vi "ReadVolumePoint.vi"(10 "Scan Settings":T1, 11 "Command":enum16{"Init", "Get Point"}(ring)) -> (2 "Finished":bool, 3 "Point":cluster{"X":i32, "Y":i32, "Z":i32})   [LabVIEW 2012]
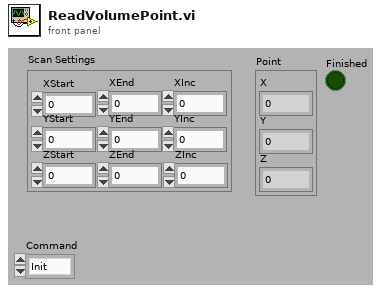
[diagram p1: front panel]
types:
  T1 = cluster{"XStart":i32, "XEnd":i32, "XInc":i32, "YStart":i32, "YEnd":i32, "YInc":i32, "ZStart":i32, "ZEnd":i32, "ZInc":i32}
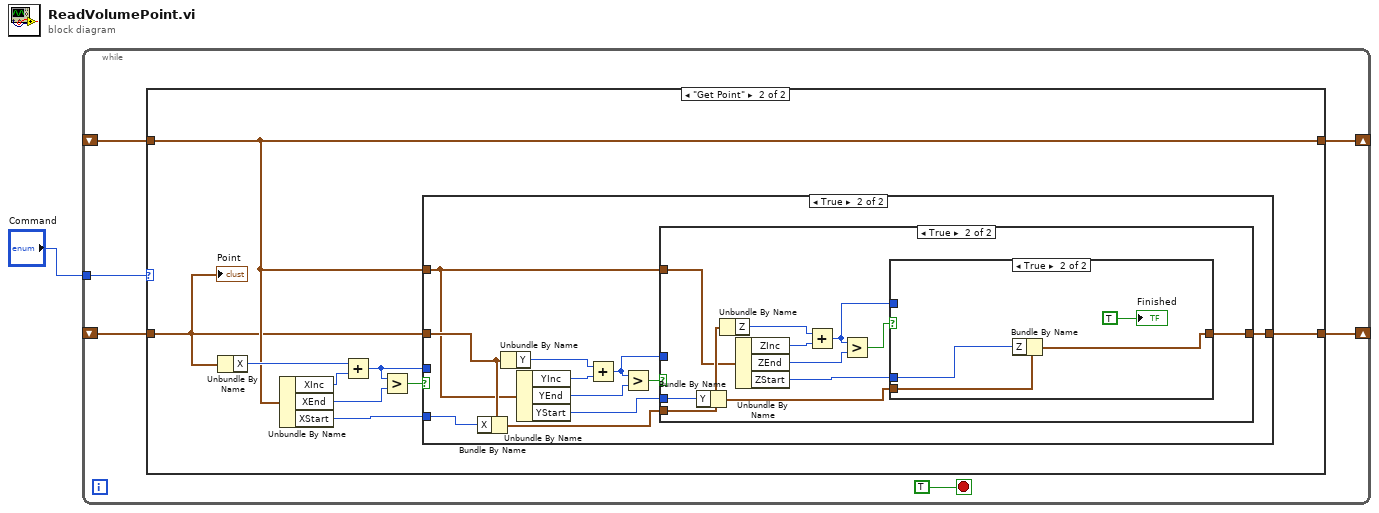
[diagram p0: block diagram]
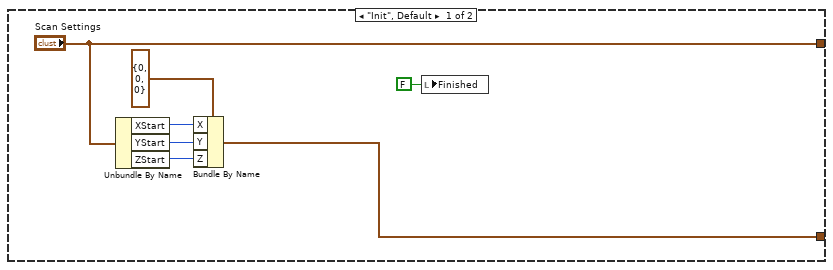
[diagram p2: hidden frame]
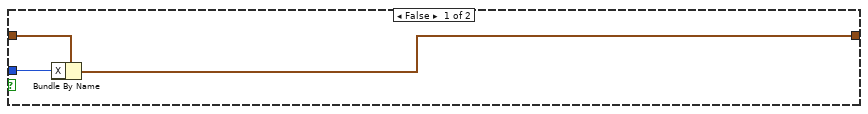
[diagram p3: hidden frame]
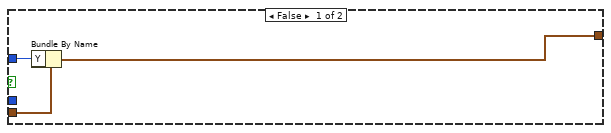
[diagram p4: hidden frame]
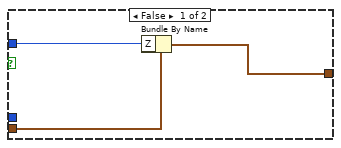
[diagram p5: hidden frame]
diagram:
  n1 = while {
    tunnel: "Command" -> [w6]
    shift-right: [w5] -> _
    shift-left: _ -> [w4]
    shift-right: [w2] -> _
    shift-left: _ -> [w3]
    stop <- TRUE stop-if-true
    n2 = case shown="\"Get Point\"" w6 {
      tunnel: ["Scan Settings" w19] -> w5
      tunnel: w4 -> [_ w19]
      tunnel: w3 -> [_ w17]
      tunnel: [w10 w16] -> w2
      frame "Init", Default {
        n3 = Unbundle By Name("Scan Settings") -> ("XStart"=w13:i32, "YStart"=w12:i32, "ZStart"=w11:i32)
        n4 = Bundle By Name(cluster=cluster{"X":i32, "Y":i32, "Z":i32} {"X"=0, "Y"=0, "Z"=0} ("Point"), "X"=w13, "Y"=w12, "Z"=w11) -> (w10:cluster{"X":i32, "Y":i32, "Z":i32})
        n5 = local write "Finished"(FALSE ("Finished")) -> ()
      }
      frame "Get Point" {
        n6 = Unbundle By Name(w17) -> ("X"=w23:i32)
        n7 = Unbundle By Name(w19) -> ("XInc"=w22:i32, "XEnd"=w21:i32, "XStart"=w15:i32)
        n8 = Add(x=w23, y=w22) -> (x+y=w18:i32)
        n9 = Greater?(x=w18, y=w21) -> (0:w20:bool)
        n10 = case shown="True" w20 {
          tunnel: w19 -> [_ w28]
          tunnel: w18 -> [w25 _]
          tunnel: w17 -> [w26 w37]
          tunnel: [w24 w31] -> w16
          tunnel: w15 -> [_ w33]
          frame False {
            n11 = Bundle By Name(cluster=w26, "X"=w25) -> (w24:cluster{"X":i32, "Y":i32, "Z":i32})
          }
          frame True {
            n12 = Bundle By Name(cluster=w37, "X"=w33) -> (w32:cluster{"X":i32, "Y":i32, "Z":i32})
            n13 = Unbundle By Name(w37) -> ("Y"=w29:i32)
            n14 = Unbundle By Name(w28) -> ("YInc"=w36:i32, "YEnd"=w35:i32, "YStart"=w30:i32)
            n15 = Add(x=w29, y=w36) -> (x+y=w27:i32)
            n16 = Greater?(x=w27, y=w35) -> (0:w34:bool)
            n17 = case shown="True" w34 {
              tunnel: w32 -> [w40 w48]
              tunnel: [w39 w42] -> w31
              tunnel: w30 -> [_ w51]
              tunnel: w27 -> [w38 _]
              tunnel: w28 -> [_ w47]
              frame False {
                n18 = Bundle By Name(cluster=w40, "Y"=w38) -> (w39:cluster{"X":i32, "Y":i32, "Z":i32})
              }
              frame True {
                n19 = Bundle By Name(cluster=w48, "Y"=w51) -> (w45:cluster{"X":i32, "Y":i32, "Z":i32})
                n20 = Unbundle By Name(w48) -> ("Z"=w43:i32)
                n21 = Unbundle By Name(w47) -> ("ZInc"=w50:i32, "ZEnd"=w49:i32, "ZStart"=w44:i32)
                n22 = Add(x=w43, y=w50) -> (x+y=w41:i32)
                n23 = Greater?(x=w41, y=w49) -> (0:w46:bool)
                n24 = case shown="True" w46 {
                  tunnel: w45 -> [w54 w58]
                  tunnel: w44 -> [_ w57]
                  tunnel: w41 -> [w53 _]
                  tunnel: [w52 w56] -> w42
                  frame False {
                    n25 = Bundle By Name(cluster=w54, "Z"=w53) -> (w52:cluster{"X":i32, "Y":i32, "Z":i32})
                  }
                  frame True {
                    n26 = Bundle By Name(cluster=w58, "Z"=w57) -> (w56:cluster{"X":i32, "Y":i32, "Z":i32})
                    "Finished" <- TRUE ("Finished")
                  }
                }
              }
            }
          }
        }
        "Point" <- w17
      }
    }
  }
